vi "test -- sweeper -- V2.vi"(1 "MFLI controller action":T1=enum."Scan frequency", 13 "delay (msec)":i64=3) -> ()   [LabVIEW 2017]
uses:
  MFLI controller action.ctl
  sweep parameters.ctl
  cursor winow.ctl
  <vilib>/event_ctls.llb/eventvkey.ctl
  cursor window action.ctl
  publisher action.ctl
panel:
  out "size":i32
  out "center freq (Hz) 2":dbl=1204.0368684802743
  out "window  (Hz) 2":dbl=985.4468417621292
  out "left freq (Hz) 2":dbl=711.3134475992097
  out "right freq (Hz) 2":dbl=1696.760289361339
  in  "all 3":enum32{"all", "other", "other 2"}(tab)
  out "Plot: complex plane - filter":cluster{dbl[], dbl[]}[](graph)
  in  "Stop!":bool
  in  "N":i64=200
  in  "scan type":enum16{"linear", "arctan"}(ring)
  out "right freq (Hz)":dbl=8.26461485679713
  out "left freq (Hz)":dbl=-8.969831627629043
  out "window  (Hz)":dbl=17.234446484426172
  out "center freq (Hz)":dbl=-0.35260838541595674
  in  "sweep parameters":T2={"scan type"=enum."linear", "N"=200, "cursor window"={"left"=2378.60310421286, "right "=2421.6740576496672, "center"=2421.6740576496672, "window"=2421.6740576496672, "cursors"=[], "relative"=0, "absolute"=0, "fixed vertical offset"=2421.6740576496672, "vertical offset"=2421.6740576496672, "skew"=2421.6740576496672, "default window frac"=2421.6740576496672, "kind"=enum."skewed", "skew.left"=2421.6740576496672, "skew.right"=2421.6740576496672, "Plot ref"=refnum, "wing order"=enum."back"}}
  out "VKey":T4=enum."Cmd"
  out "Char":i16
  in  "cursor bracket: fit boundaries":T3={"left"=711.3134475992097, "right "=1696.760289361339, "center"=1204.0368684802743, "window"=985.4468417621292, "cursors"=[0, 1, 2], "relative"=2, "absolute"=2, "fixed vertical offset"=0.0, "vertical offset"=0.0, "skew"=0.0, "default window frac"=0.1, "kind"=enum."symmetric", "skew.left"=0.5, "skew.right"=0.5, "Plot ref"=refnum, "wing order"=enum."forw"}
  in  "all":enum32{"all", "other"}(tab)
  out "Plot: hist":cluster{"all rows":dbl[], "all rows":dbl[]}[](graph)
  out "dev out":cdb=-0.0006525009086557267-6.386367654802008e-07i format="%#_10f"
  out "freq":dbl=5.0 format="%#_10f"
  out "scan progress":i32(slide)=162 min=0 max=2000 scale=0.0..2000.0
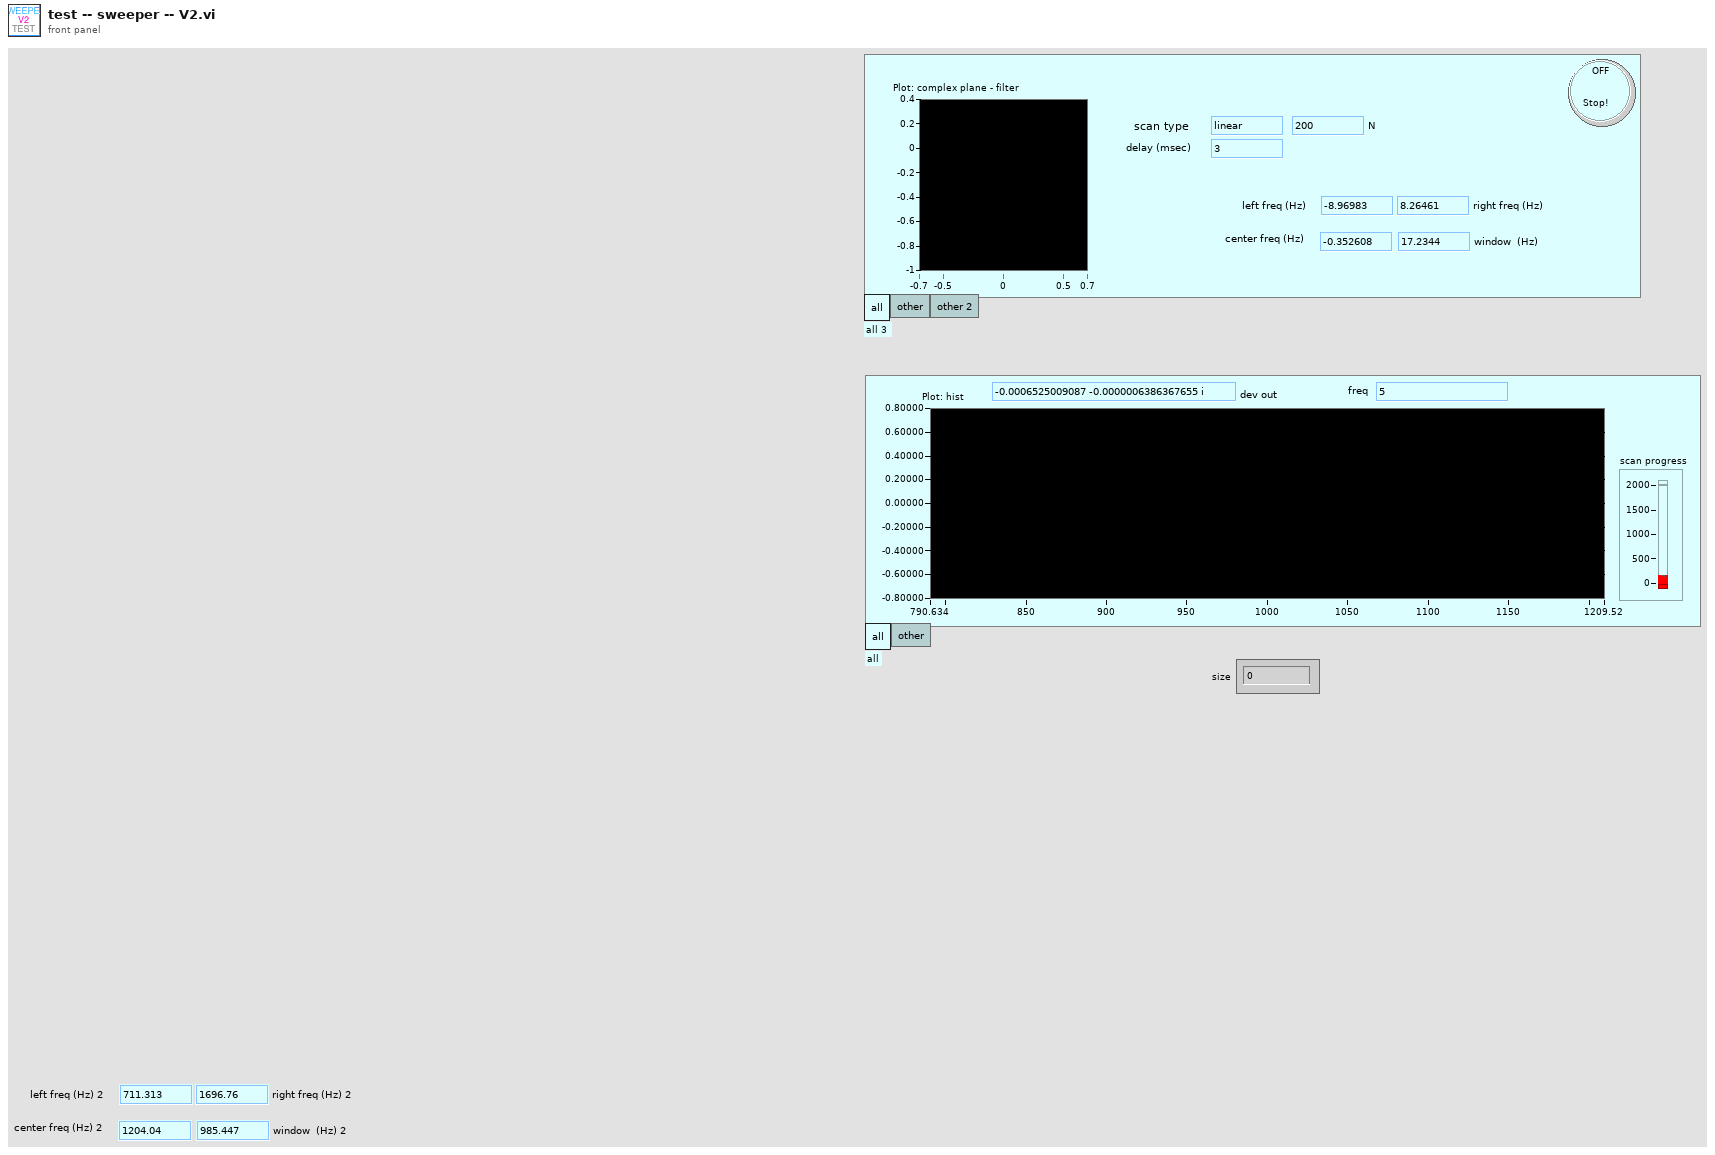
[diagram p1: front panel]
types:
  T1 = typedef "MFLI controller action.ctl" = enum16{"Initialize", "Scan frequency", "open", "close", "read", "circle PLL"}
  T2 = typedef "sweep parameters.ctl" = cluster{"scan type":enum16{"linear", "arctan"}, "N":i64, "cursor window":T3}
  T3 = typedef "cursor winow.ctl" = cluster{"left":dbl, "right ":dbl, "center":dbl, "window":dbl, "cursors":i32[], "relative":i32, "absolute":i32, "fixed vertical offset":dbl, "vertical offset":dbl, "skew":dbl, "default window frac":dbl, "kind":enum16{"symmetric", "skewed", "fancy"}, "skew.left":dbl, "skew.right":dbl, "Plot ref":refnum<vi>, "wing order":enum16{"forw", "back"}}
  T4 = typedef "eventvkey.ctl" = enum16{"ASCII", "Enter", "Return", "Shift", "Ctrl", "Alt", "Cmd", "Opt", "Caps", "NumLock", "Clear", "Break", "Up", "Down", "Left", "Right", "Insert", "Delete", "Home", "End", "PageUp", "PageDown", "Escape", "Help", "Pause", "ScrollLock", "F1", "F2", "F3", "F4", "F5", "F6", "F7", "F8", "F9", "F10", "F11", "F12", "F13", "F14", "F15", "F16", "F17", "F18", "F19", "F20", "F21", "F22", "F23", "F24", "Play", "VolumeUp", "VolumeDown", "Mute", "Two Byte Char"}
  T5 = typedef "cursor window action.ctl" = enum16{"balance", "h. offset change", "cursor moves", "change center", "change window", "init", "check", "reset", "set y to middle", "idle", "-write all Y", "-write left.X", "-write center.X", "-write right.X", "-write all X", "-change center", "-change window", "-change skew", "-read cursor 2", "-read cursor 1", "-read cursor 0", "-read all cursors", "-reset", "-read plot scale", "-set y to middle", "-Q: center.Y is visible", "-Q: window is visible", "-parse center.Y", "-right left from center", "-left move", "-right move", "-set center.Y", "-empty", "-set cursors to default", "-check", "-write center.Y", "-copy cursor 1", "-copy cursor 0", "-copy cursor 2", "move right", "move left", "shrink", "broaden", "skew up", "skew down", "-write plot scale", "zoom X", "change cen&win", "zoom to all data", "color--red", "color--green", "color--yellow", "read", "zoom out", "zoom in", "slide right", "slide left"}
  T6 = typedef "publisher action.ctl" = enum16{"set", "get"}
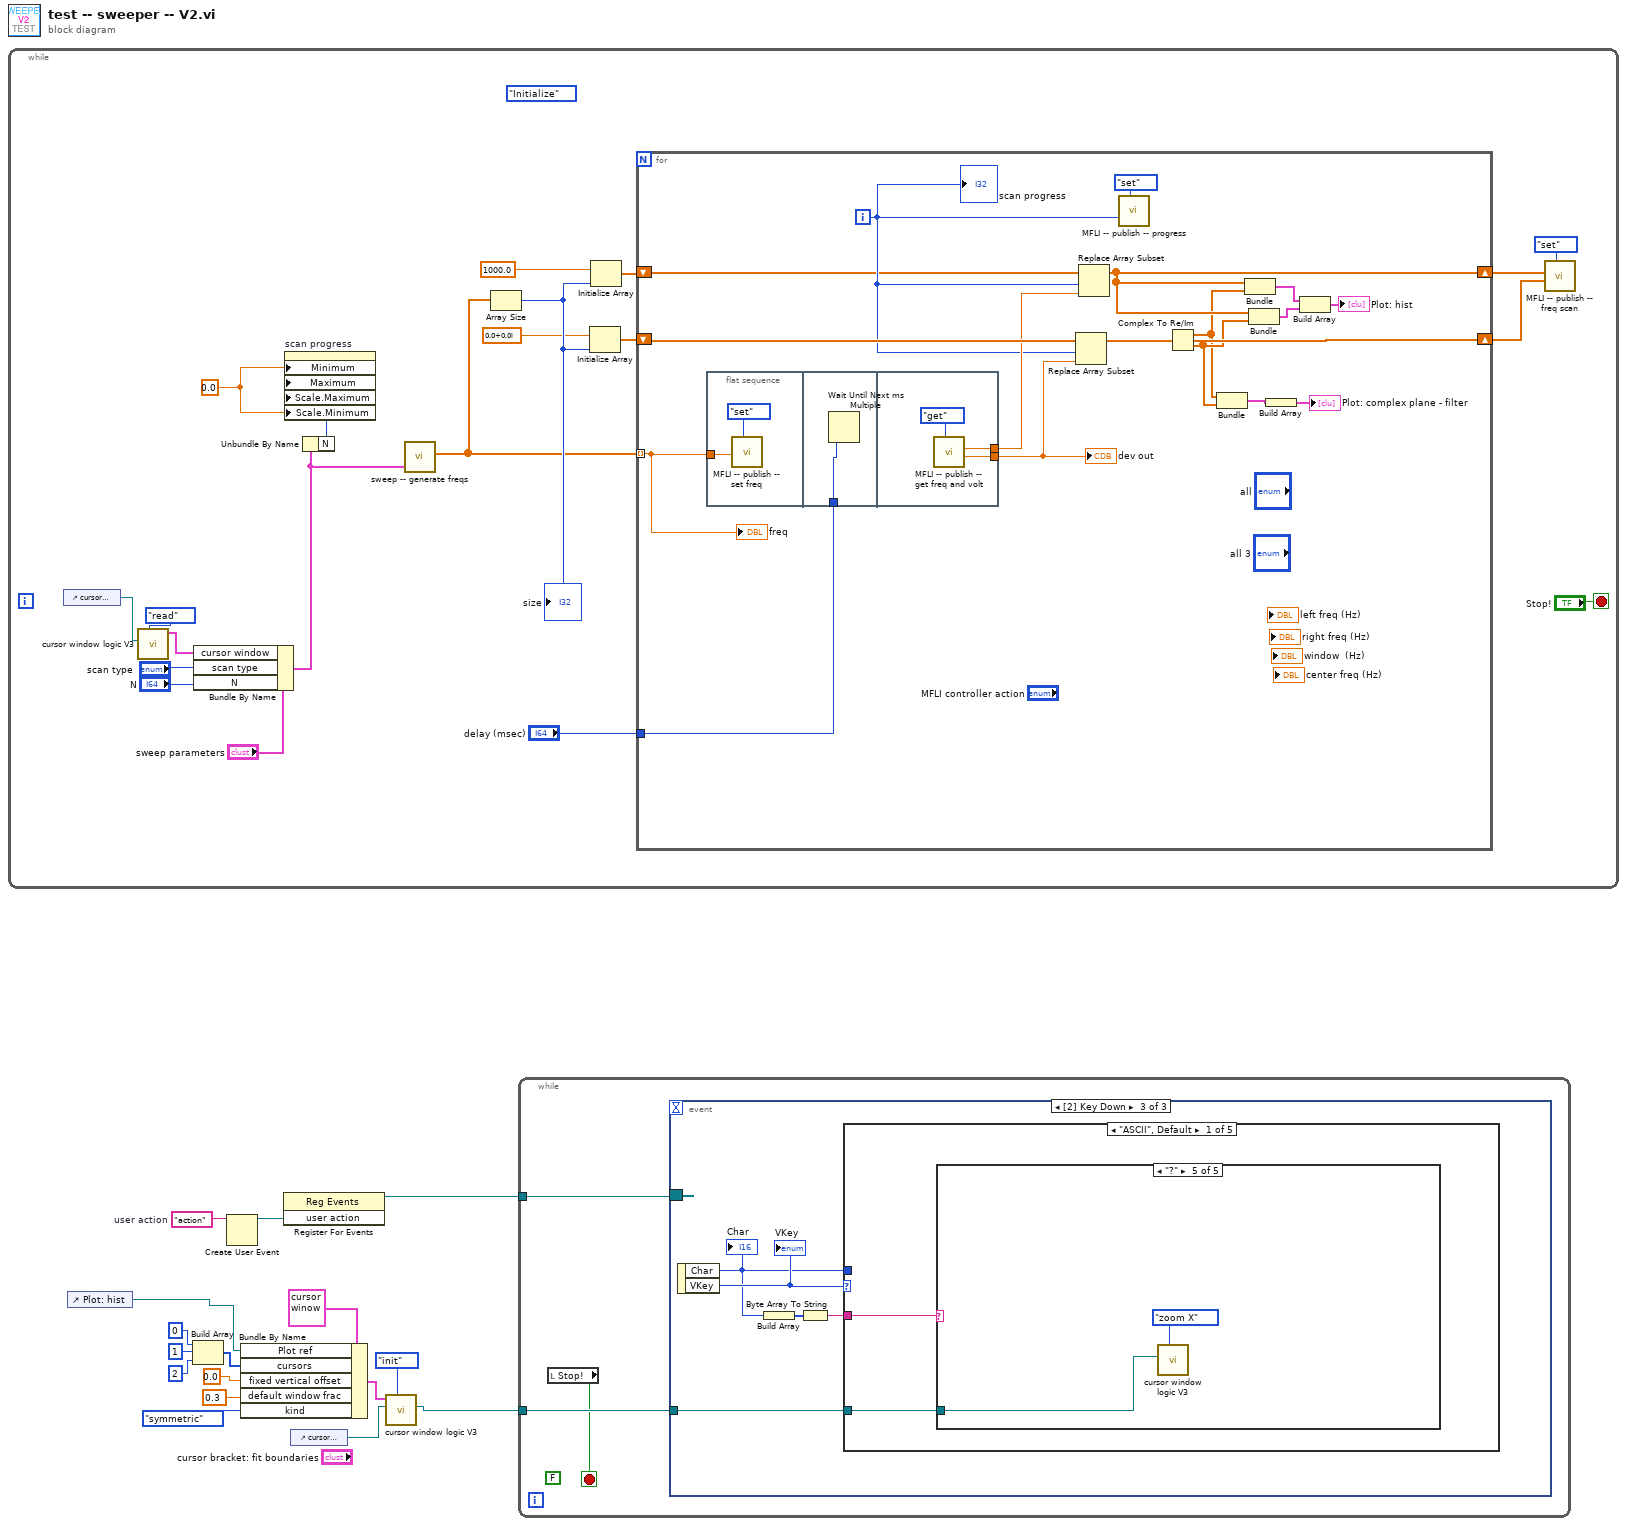
[diagram p0: block diagram]
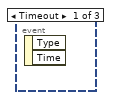
[diagram p2: hidden frame]
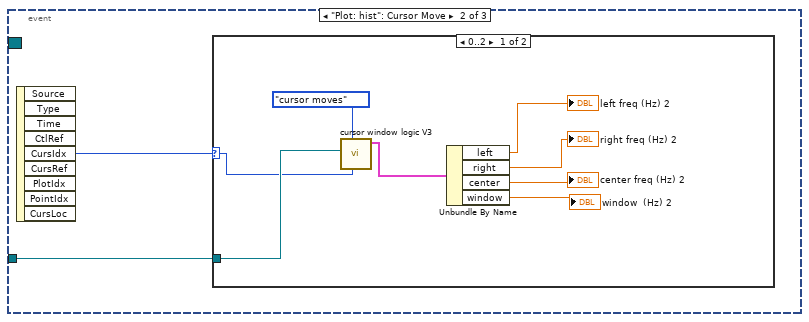
[diagram p3: hidden frame]
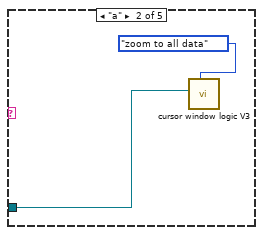
[diagram p6: hidden frame]
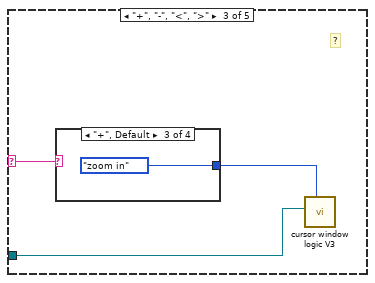
[diagram p7: hidden frame]
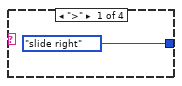
[diagram p8: hidden frame]
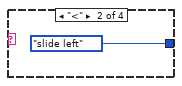
[diagram p9: hidden frame]
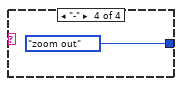
[diagram p10: hidden frame]
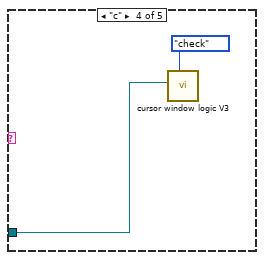
[diagram p11: hidden frame]
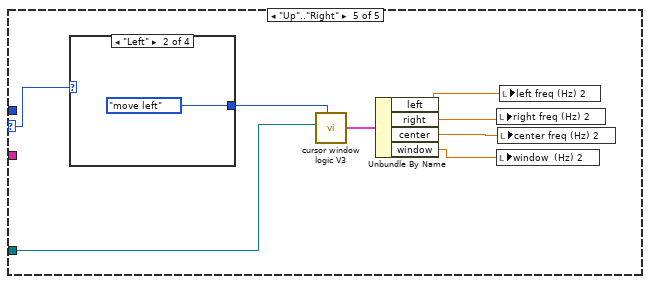
[diagram p15: hidden frame]
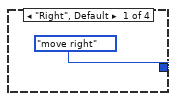
[diagram p16: hidden frame]
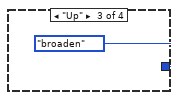
[diagram p17: hidden frame]
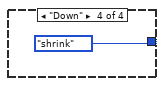
[diagram p18: hidden frame]
diagram:
  w14 = "action"  # user action
  n1 = while {
    stop <- "Stop!" stop-if-true
    (unwired) MFLI_controller_action."Initialize" ("MFLI controller action")
    w35 = 0.0 ("Data Entry Limits:Minimum")
    n2 = control-ref of="cursor bracket: fit boundaries"() -> (w26:refnum<vi>)
    n3 = call "cursor window logic V3.vi"("cursor window action"=cursor_window_action."read", "cursor window in"=w26) -> ("cursor window out"=w29:T3)  [unwired: 8 in, 1 out]
    n4 = Bundle By Name(cluster="sweep parameters", "cursor window"=w29, "scan type"="scan type", "N"="N") -> (w24:T2)
    n5 = Unbundle By Name(w24) -> ("N"=w23:i64)
    n6 = property on="scan progress" class="Slide (strict)"("Minimum"=w35, "Maximum"=w23, "Scale.Maximum"=w23, "Scale.Minimum"=w35) -> ()  [unwired: 2 in, 2 out]
    n7 = call "sweep -- generate freqs.vi"("sweep parameters"=w24) -> ("Array"=w17:dbl[])  [unwired: 10 in]
    n8 = Array Size(array=w17) -> (size(s)=w22:i32)
    "size" <- w22
    n9 = Initialize Array(cdb 0.0+0.0i ("Data Entry Limits:Minimum"), w22) -> (w18:cdb[])
    n10 = Initialize Array(1000.0 ("Data Entry Limits:Minimum"), w22) -> (w19:dbl[])
    n11 = for {
      tunnel: w17 -> [w38] mode=indexing
      tunnel: "delay (msec)" -> [w53]
      shift-right: [w44] -> w31
      shift-left: w18 -> [w51]
      shift-right: [w43] -> w32
      shift-left: w19 -> [w48]
      i -> [w49]
      n12 = flat-sequence {
        tunnel: w38 -> [w55]
        tunnel: w53 -> [w56]
        tunnel: [w58] -> w37
        tunnel: [w57] -> w50
        frame #0 {
          n13 = call "MFLI -- publish -- set freq.vi"("publisher action"=publisher_action."set", "freq IN (Hz)"=w55) -> ()  [unwired: 9 in, 1 out]
        }
        frame #1 {
          n14 = Wait Until Next ms Multiple(millisecond multiple=w56) -> ()  [unwired: 1 out]
        }
        frame #2 {
          n15 = call "MFLI -- publish -- get freq and volt.vi"("publisher action"=publisher_action."get") -> ("Voltage out (V)"=w58:cdb, "freq out (Hz)"=w57:dbl)  [unwired: 9 in]
        }
      }
      n16 = Replace Array Subset(array=w51, new element=w37, index=w49) -> (w44:cdb[])
      n17 = Replace Array Subset(array=w48, new element=w50, index=w49) -> (w43:dbl[])
      n18 = call "MFLI -- publish -- progress.vi"("publisher action"=publisher_action."set", "num"=w49) -> ()  [unwired: 9 in, 1 out]
      n19 = Complex To Re/Im(x + iy=w44) -> (x=w41:dbl[], y=w42:dbl[])
      n20 = Bundle(w41, w42) -> (w40:cluster{dbl[], dbl[]})  [unwired: 1 in]
      n21 = Bundle(w43, w41) -> (w47:cluster{dbl[], dbl[]})  [unwired: 1 in]
      n22 = Bundle(w43, w42) -> (w46:cluster{dbl[], dbl[]})  [unwired: 1 in]
      n23 = Build Array(w40) -> (→"Plot: complex plane - filter":cluster{dbl[], dbl[]}[])
      n24 = Build Array(w47, w46) -> (→"Plot: hist":cluster{dbl[], dbl[]}[])
      "scan progress" <- w49
      "freq" <- w38
      "dev out" <- w37
    }
    n25 = call "MFLI -- publish -- freq scan.vi"("publisher action"=publisher_action."set", "Voltage IN (V)"=w31, "Freq IN (Hz)"=w32) -> ()  [unwired: 7 in, 2 out]
  }
  n26 = control-ref of="Plot: hist"() -> (w1:refnum<vi>)
  n27 = Build Array(0, 1, 2) -> (w2:i32[])
  n28 = Create User Event(user event datatype=w14) -> (user event=w15:refnum<user-event>)  [unwired: 1 in, 1 out]
  n29 = Bundle By Name(cluster=T3 {"left"=0.0, "right "=0.0, "center"=0.0, "window"=0.0, "cursors"=[], "relative"=0, "absolute"=0, "fixed vertical offset"=0.0, "vertical offset"=0.0, "skew"=0.0, "default window frac"=0.0, "kind"=enum."symmetric", "skew.left"=0.0, "skew.right"=0.0, "Plot ref"=refnum, "wing order"=enum."forw"} ("cursor bracket: All, data window"), "Plot ref"=w1, "cursors"=w2, "fixed vertical offset"=0.0, "default window frac"=0.3 ("fixed vertical offset"), "kind"=enum16{"symmetric", "skewed", "fancy"}."symmetric") -> (w10:T3)
  n30 = register-events(w15) -> (reference out=w13:refnum<event-registration>)  [unwired: 2 in, 1 out]
  n31 = control-ref of="cursor bracket: fit boundaries"() -> (w12:refnum<vi>)
  n32 = call "cursor window logic V3.vi"("cursor window action"=cursor_window_action."init", "cursor window in"=w12, "cursor window init"=w10) -> ("cursor window out"=w16:refnum<vi>)  [unwired: 7 in, 1 out]
  n33 = while {
    tunnel: w13 -> [w62]
    tunnel: w16 -> [w61]
    stop <- w60 stop-if-true
    (unwired) FALSE
    n34 = local read "Stop!"() -> (w60:bool)
    n35 = event shown="[2] Key Down" {
      selector: w62 -> [_ _ _]
      dyn-events: _ -> [_ _ _]
      timeout: _ -> [_ _ _]
      tunnel: w61 -> [_ w64 w73]
      event Timeout {
        n36 = event-data() -> ()  [unwired: 1 in, 2 out]
      }
      event "Plot: hist": Cursor Move {
        n37 = event-data() -> ("CursIdx"=w63:i32)  [unwired: 1 in, 8 out]
        n38 = case shown="0..2" w63 {
          selector: w63 -> [w70 _]
          tunnel: w64 -> [w72 _]
          frame 0..2 {
            n39 = call "cursor window logic V3.vi"("CursIdx"=w70, "cursor window action"=cursor_window_action."cursor moves", "cursor window in"=w72) -> ("cursor window out"=w69:T3)  [unwired: 7 in, 1 out]
            n40 = Unbundle By Name(w69) -> ("left"=→"left freq (Hz) 2":dbl, "right"=→"right freq (Hz) 2":dbl, "center"=→"center freq (Hz) 2":dbl, "window"=→"window  (Hz) 2":dbl)
          }
          frame 3, Default {
          }
        }
      }
      event Key Down {
        n41 = event-data() -> ("Char"=w75:i16, "VKey"=w77:T4)  [unwired: 1 in]
        "Char" <- w75
        "VKey" <- w77
        n42 = Build Array(w75) -> (w76:i16[])
        n43 = Byte Array To String(unsigned byte array=w76) -> (string=w74:string)
        n44 = case shown="\"ASCII\", Default" w77 {
          selector: w77 -> [_ _ _ _ w100]
          tunnel: w75 -> [_ _ _ _ _]
          tunnel: w74 -> [w79 _ _ _ _]
          tunnel: w73 -> [w78 _ _ _ w93]
          frame "ASCII", Default {
            n45 = case shown="\"?\"" w79 {
              selector: w79 -> [_ _ w83 _ _]
              tunnel: w78 -> [_ w80 w84 w89 w91]
              frame "0", Default {
              }
              frame "a" {
                n46 = call "cursor window logic V3.vi"("cursor window action"=cursor_window_action."zoom to all data", "cursor window in"=w80) -> ()  [unwired: 8 in, 2 out]
              }
              frame "+", "-", "<", ">" {
                # "?"
                n47 = case shown="\"+\", Default" w83 {
                  tunnel: [cursor_window_action."slide right" ("cursor window action") cursor_window_action."slide left" ("cursor window action") cursor_window_action."zoom in" ("cursor window action") cursor_window_action."zoom out" ("cursor window action")] -> w82
                  frame ">" {
                  }
                  frame "<" {
                  }
                  frame "+", Default {
                  }
                  frame "-" {
                  }
                }
                n48 = call "cursor window logic V3.vi"("cursor window action"=w82, "cursor window in"=w84) -> ()  [unwired: 8 in, 2 out]
              }
              frame "c" {
                n49 = call "cursor window logic V3.vi"("cursor window action"=cursor_window_action."check", "cursor window in"=w89) -> ()  [unwired: 8 in, 2 out]
              }
              frame "?" {
                n50 = call "cursor window logic V3.vi"("cursor window action"=cursor_window_action."zoom X", "cursor window in"=w91) -> ()  [unwired: 8 in, 2 out]
              }
            }
          }
          frame "Escape" {
          }
          frame "PageUp" {
          }
          frame "PageDown" {
          }
          frame "Up".."Right" {
            n51 = case shown="\"Left\"" w100 {
              tunnel: [cursor_window_action."move right" ("cursor window action") cursor_window_action."move left" ("cursor window action") cursor_window_action."broaden" ("cursor window action") cursor_window_action."shrink" ("cursor window action")] -> w95
              frame "Right", Default {
              }
              frame "Left" {
              }
              frame "Up" {
              }
              frame "Down" {
              }
            }
            n52 = call "cursor window logic V3.vi"("cursor window action"=w95, "cursor window in"=w93) -> ("cursor window out"=w94:T3)  [unwired: 8 in, 1 out]
            n53 = Unbundle By Name(w94) -> ("left"=w99:dbl, "right"=w98:dbl, "center"=w97:dbl, "window"=w96:dbl)
            n54 = local write "right freq (Hz) 2"(w98) -> ()
            n55 = local write "window  (Hz) 2"(w96) -> ()
            n56 = local write "center freq (Hz) 2"(w97) -> ()
            n57 = local write "left freq (Hz) 2"(w99) -> ()
          }
        }
      }
    }
  }
